vi "Control_Tablero.vi"() -> ()   [LabVIEW 2024]
panel:
  out "Meter":dbl(knob) scale=0.0..10.0
  in  "stop":bool
  in  "Activación Eje":bool
  out "Estado Eje":bool
  in  "Habilitar Eje":bool
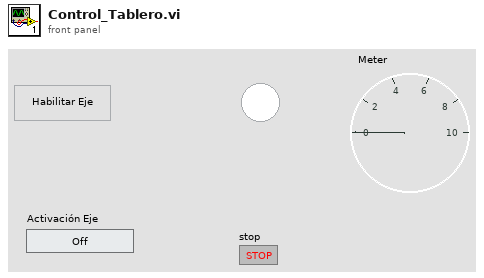
[diagram p1: front panel]
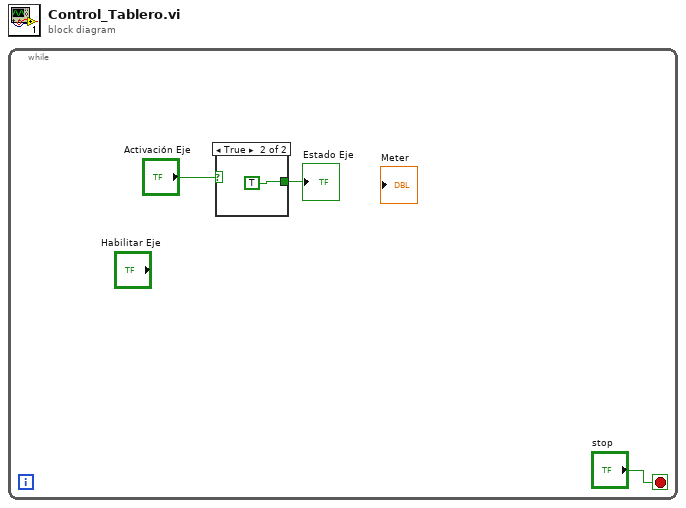
[diagram p0: block diagram]
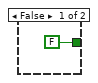
[diagram p2: hidden frame]
diagram:
  n1 = while {
    stop <- "stop" stop-if-true
    n2 = case shown="True" "Activación Eje" {
      tunnel: [FALSE TRUE] -> w2
      frame False {
      }
      frame True {
      }
    }
    "Estado Eje" <- w2
  }
